vi "Validation Class.vi"() -> ()   [LabVIEW 2020, in "Library Instrument & Equipement.lvlib" / "Library FireBase.lvlib" / "Firebase Find_Batch_Fct_SN.lvclass"]
uses:
  Firebase Find_Batch_Fct_SN.lvclass
  C:/Users/ngarcin/OneDrive - Altyor/Standard TB/Class/Firebase/Source/Firebase Driver/Firebase Driver.lvclass
  Firebase Find_Batch_Fct_SN.lvclass/Firebase Find_Batch_Fct_SN.ctl
panel:
  out "Read_Data":T1(array[cluster])
  out "sortie d'erreur":errorcluster
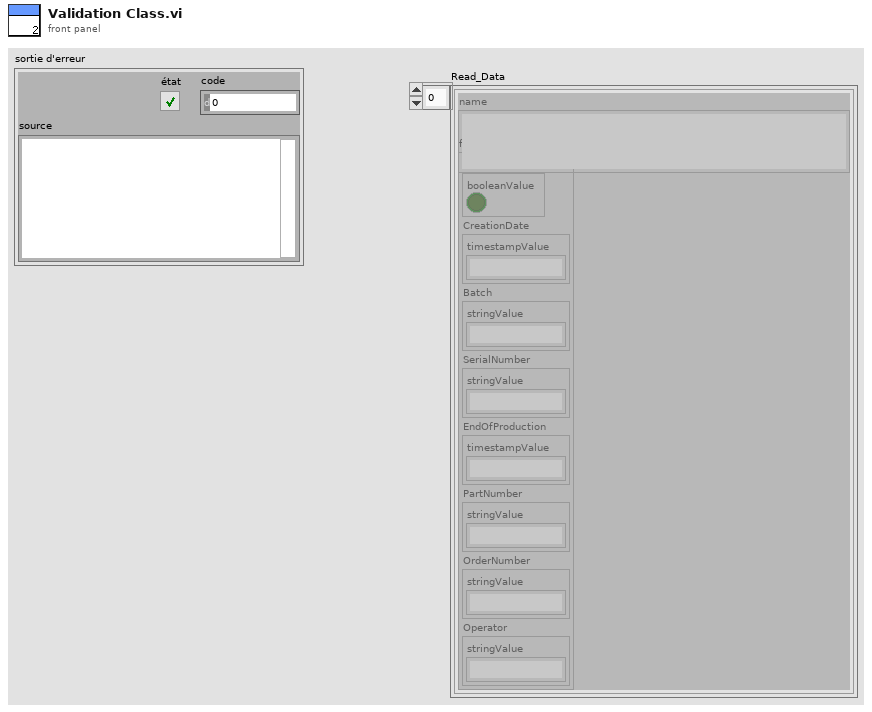
[diagram p1: front panel]
types:
  T1 = cluster{"name":string, "fields":cluster{"Result":cluster{"booleanValue":bool}, "CreationDate":cluster{"timestampValue":string}, "Batch":cluster{"stringValue":string}, "SerialNumber":cluster{"stringValue":string}, "EndOfProduction":cluster{"timestampValue":string}, "PartNumber":cluster{"stringValue":string}, "OrderNumber":cluster{"stringValue":string}, "Operator":cluster{"stringValue":string}}}[]
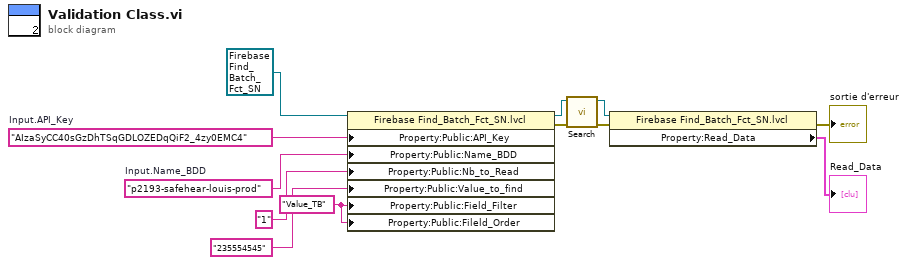
[diagram p0: block diagram]
diagram:
  w1 = "Value_TB" ("Field_Filter")
  w11 = "AIzaSyCC40sGzDhTSqGDLOZEDqQiF2_4zy0EMC4"  # Input.API_Key
  w10 = "p2193-safehear-louis-prod"  # Input.Name_BDD
  n1 = property class="Firebase Find_Batch_Fct_SN.lvcl"(reference=refnum<class "Firebase Find_Batch_Fct_SN.lvclass"> refnum ("Build Library FireBase.lvlib:Firebase AssembledProducts.lvclass"), "Property:Public:API_Key"=w11, "Property:Public:Name_BDD"=w10, "Property:Public:Nb_to_Read"="1" ("Nb_to_Read"), "Property:Public:Value_to_find"="235554545" ("Value_to_find"), "Property:Public:Field_Filter"=w1, "Property:Public:Fileld_Order"=w1) -> (reference out=w8:refnum<class "Firebase Find_Batch_Fct_SN.lvclass">, error out=w7:errorcluster)  [unwired: 1 in]
  n2 = call-dynamic "Search.vi"("error in (no error)"=w7, "Firebase Benches en entrée"=w8) -> ("error out"=w5:errorcluster, "Firebase Benches en sortie"=w4:refnum<class "Firebase Find_Batch_Fct_SN.lvclass">)  [unwired: 8 in]
  n3 = property class="Firebase Find_Batch_Fct_SN.lvcl"(reference=w4, error in=w5) -> (error out=→"sortie d'erreur":errorcluster, "Property:Read_Data"=→"Read_Data":T1)  [unwired: 1 out]
